vi "c Spark Set CAN Timeout.vi"(8 "error in (no error)":errorcluster, 10 "timeoutMs":i32, 11 "handle":T1) -> (0 "error out":errorcluster, 2 "function return":T2, 3 "handle out":T1)   [LabVIEW 2023, in "REVLibDriver.lvlib"]
doc: "c_REVLib_ErrorCode c_Spark_SetCANTimeout(c_Spark_handle handle, int timeoutMs);"
uses:
  REVLibDriver.lvlib
  REVLibDriver.dll
  Custom Controls/c_Spark_handle.ctl
  subvi/RevLibError.ctl
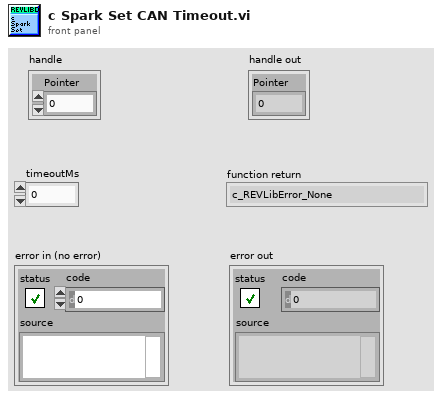
[diagram p1: front panel]
types:
  T1 = typedef "REVLibDriver.lvlib/c_Spark_handle.ctl" = cluster{"Pointer":u64}
  T2 = typedef "REVLibDriver.lvlib/RevLibError.ctl" = enum16{"c_REVLibError_None", "c_REVLibError_General", "c_REVLibError_CANTimeout", "c_REVLibError_NotImplemented", "c_REVLibError_HAL", "c_REVLibError_CantFindFirmware", "c_REVLibError_FirmwareTooOld", "c_REVLibError_FirmwareTooNew", "c_REVLibError_ParamInvalidID", "c_REVLibError_ParamMismatchType", "c_REVLibError_ParamAccessMode", "c_REVLibError_ParamInvalid", "c_REVLibError_ParamNotImplementedDeprecated", "c_REVLibError_FollowConfigMismatch", "c_REVLibError_Invalid", "c_REVLibError_SetpointOutOfRange", "c_REVLibError_Unknown", "c_REVLibError_CANDisconnected", "c_REVLibError_DuplicateCANId", "c_REVLibError_InvalidCANId", "c_REVLibError_SparkMaxDataPortAlreadyConfiguredDifferently", "c_REVLibError_SparkFlexBrushedWithoutDock", "c_REVLibError_InvalidBrushlessEncoderConfiguration", "c_REVLibError_FeedbackSensorIncompatibleWithDataPortConfig", "c_REVLibError_ParamInvalidChannel", "c_REVLibError_ParamInvalidValue", "c_REVLibError_CannotPersistParametersWhileEnabled", "c_REVLibError_NotReadyToReceiveCommand", "c_REVLibError_NumCodes"}
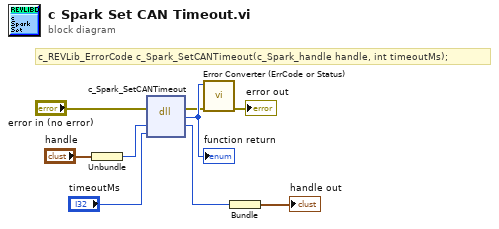
[diagram p0: block diagram]
diagram:
  # "c_REVLib_ErrorCode c_Spark_SetCANTimeout(c_Spark_handle handle, int timeoutMs);"
  n1 = Unbundle("handle") -> ("Pointer"=w2:u64)
  n2 = dll-call lib="REVLibDriver.*" fn="c_Spark_SetCANTimeout"(error in="error in (no error)", "handle"=w2, "timeoutMs"="timeoutMs") -> (error out=w4:errorcluster, "return type"=w9:u32, "handle"=w7:u64)  [unwired: 3 in, 1 out]
  "function return" <- w9
  n3 = call "Error Converter (ErrCode or Status).vi"("error in (no error)"=w4, "error code"=w9) -> ("error out"=→"error out":errorcluster)  [unwired: 9 in]
  n4 = Bundle("handle"=w7) -> (→"handle out":cluster{"handle":u64})  [unwired: 1 in]
